vi "ex7-9.vi"() -> ()   [LabVIEW 2013]
panel:
  out "element":dbl
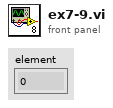
[diagram p1: front panel]
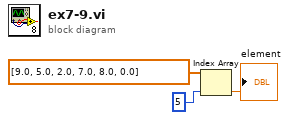
[diagram p0: block diagram]
diagram:
  n1 = Index Array(array=dbl[] [9.0, 5.0, 2.0, 7.0, 8.0, 0.0], index=5) -> (element=→"element":dbl)
